vi "GCMPlugin_GetPluginName.vi"(8 "error in (no error)":errorcluster, 11 "TemplatePlugin in":refnum<class "GCMSettingsScreen.lvclass">) -> (0 "error out":errorcluster, 2 "PluginName":string, 3 "TemplatePlugin out":refnum<class "GCMSettingsScreen.lvclass">)   [LabVIEW 2014, in "GCMSettingsScreen.lvlib" / "GCMSettingsScreen.lvclass"]
uses:
  GCMSettingsScreen.lvclass
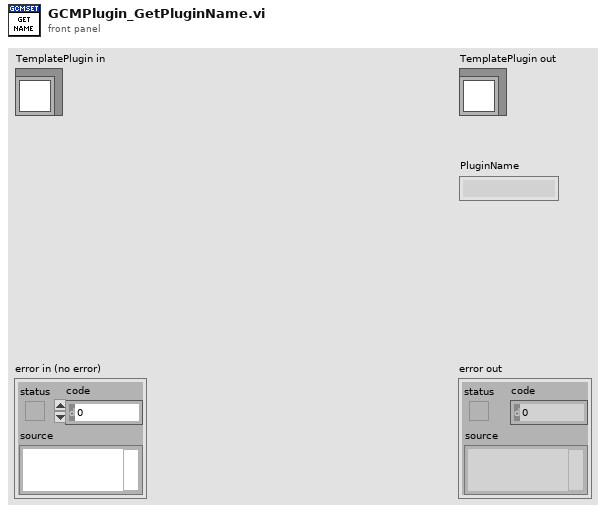
[diagram p1: front panel]
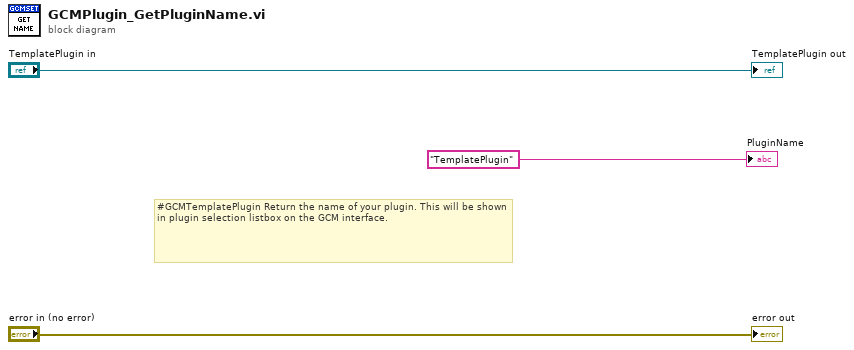
[diagram p0: block diagram]
diagram:
  # "#GCMTemplatePlugin Return the name of your plugin. This will be shown in plugin selection listbox on the GCM interface."
  "error out" <- "error in (no error)"
  "TemplatePlugin out" <- "TemplatePlugin in"
  "PluginName" <- "TemplatePlugin"
